vi "Email alert.vi"(6 "Email log file path":path=path "D:/3D FIB-SEM Files/Email Log", 7 "Send email":bool, 8 "Machine ID":string, 9 "Mail server":string, 10 "Alarm message":string, 11 "Recipents":string[](array[string])) -> ()   [LabVIEW 2018]
uses:
  <vilib>/Utility/SMTP/NI_SMTPEmail.lvlib
panel:
  in  "Hardware Configuration":T1={"SEM X coil"="SEM-X", "SEM Y coil"="SEM-Y", "FIB X coil"="FIB/ao0", "FIB Y coil"="FIB/ao1", "FIB Detector"="FIB/ai1", "SEM Detectors"="Detectors", "Det min (V)"=-10.0, "Det max (V)"=10.0, "Eanable COM"=TRUE, "COM port"="COM1", "FIB Beam blank"="FIB/port0/line0", "FIB Ext Scan"="FIB/port0/line1", "Det. FIB-NI auto switch"="FIB/port0/line2", "Post #1up"="Deflector/ao0", "Post #1down"="Deflector/ao1", "Post #2up"="Deflector/ao2", "Post #2down"="Deflector/ao3", "Machine Type"=0, "FIB Faraday Cup"="FIB/ai3", "Configuration file"=path "D:/Feiss.ini", "SEM Max FOV (um)"=198.5, "Machine ID"="Feiss2/Merlin-4238", "Save config file"=FALSE} {"Machine Type" items=["Feiss", "NVision"]}
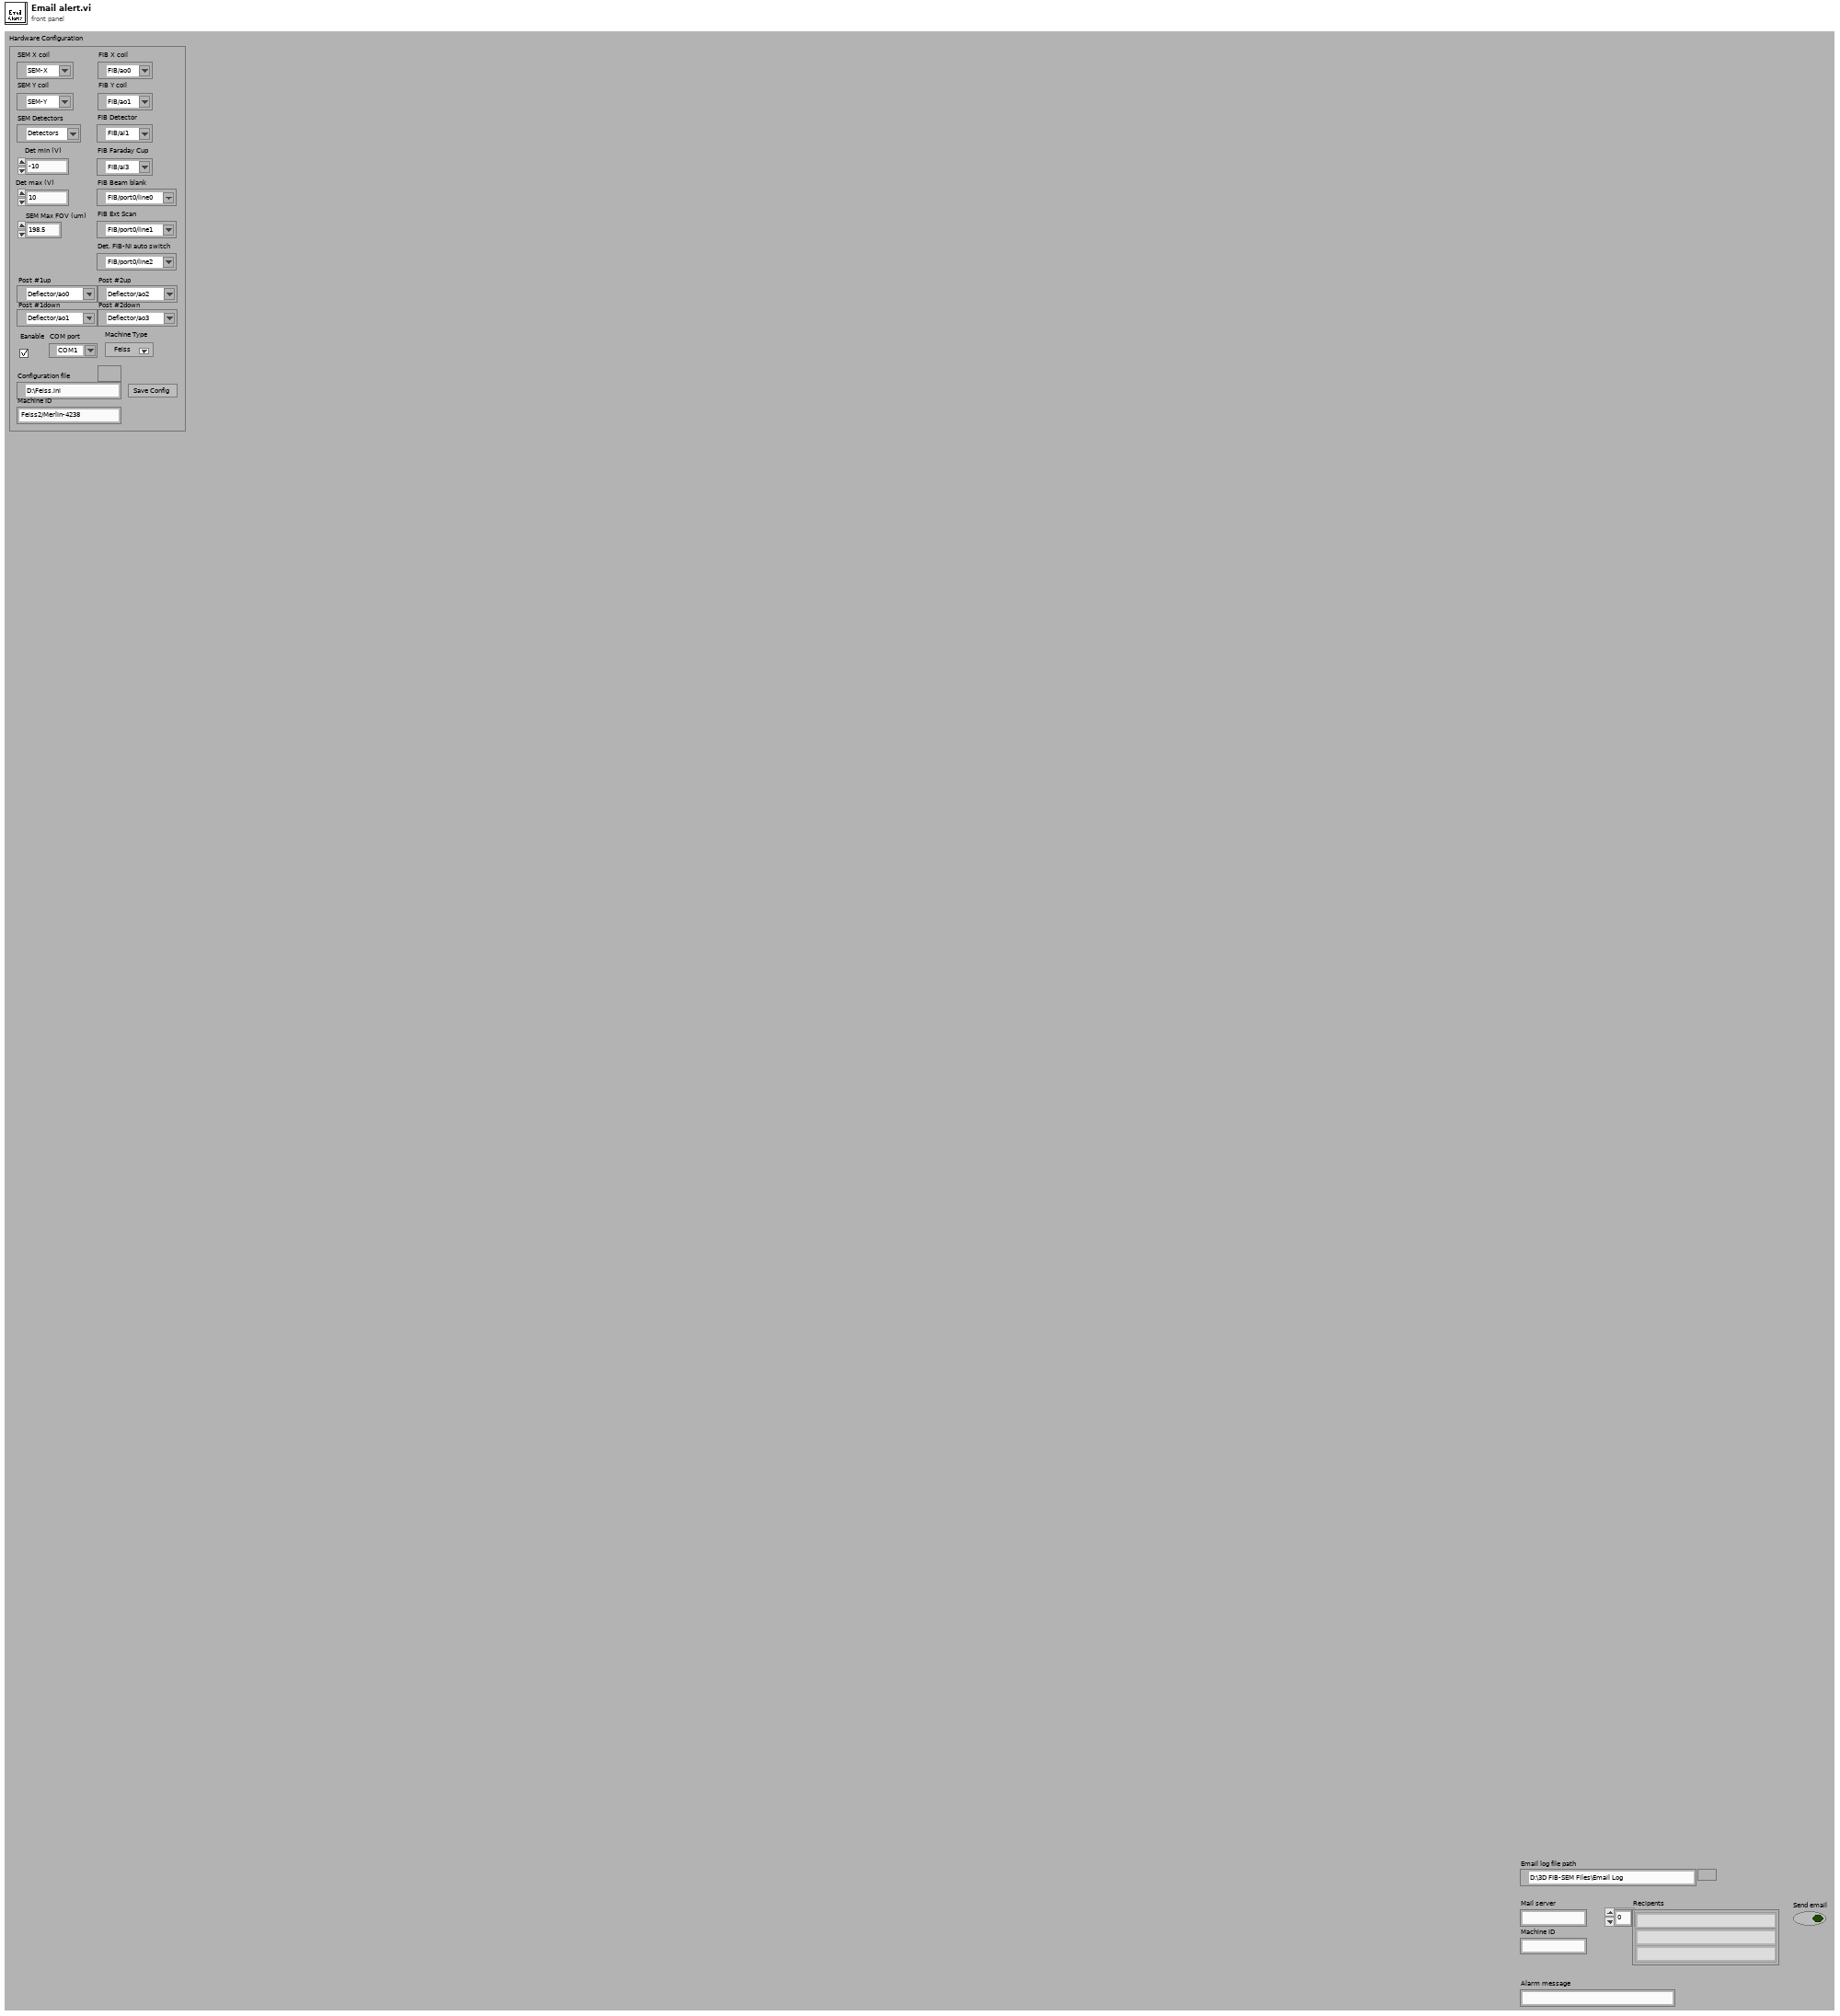
[diagram p1: front panel]
types:
  T1 = cluster{"SEM X coil":refnum<k15>, "SEM Y coil":refnum<k15>, "FIB X coil":tag, "FIB Y coil":tag, "FIB Detector":tag, "SEM Detectors":refnum<k15>, "Det min (V)":dbl, "Det max (V)":dbl, "Eanable COM":bool, "COM port":refnum<visa-resource-name>, "FIB Beam blank":tag, "FIB Ext Scan":tag, "Det. FIB-NI auto switch":tag, "Post #1up":tag, "Post #1down":tag, "Post #2up":tag, "Post #2down":tag, "Machine Type":u8, "FIB Faraday Cup":tag, "Configuration file":path, "SEM Max FOV (um)":dbl, "Machine ID":string, "Save config file":bool}
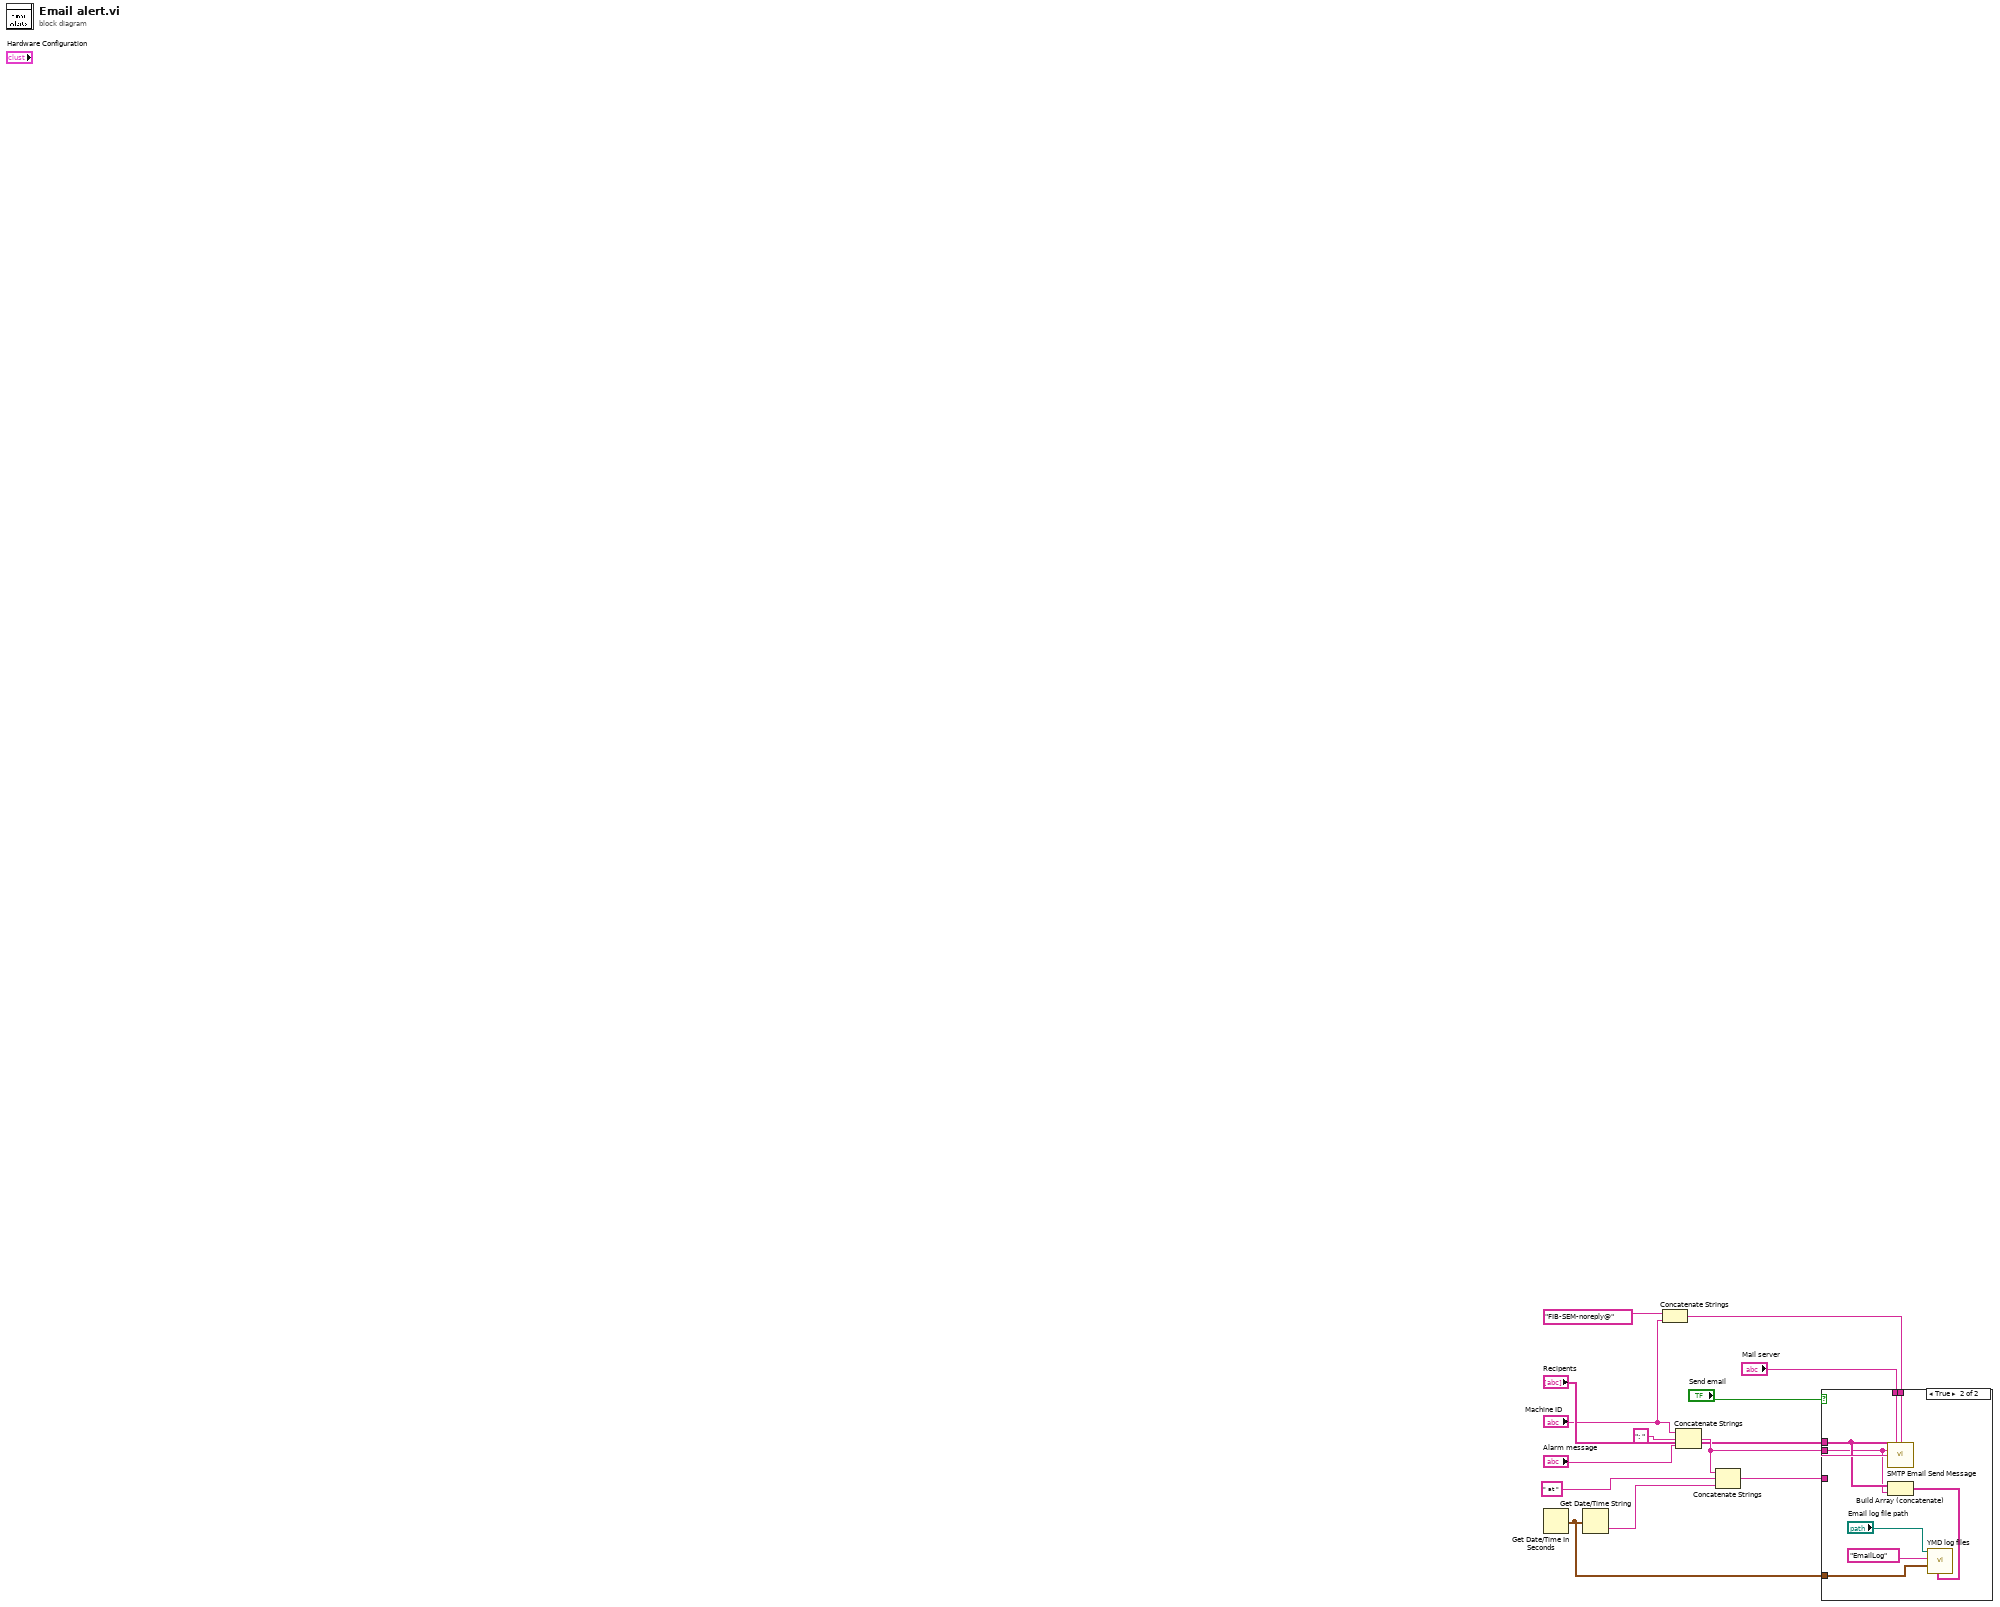
[diagram p0: block diagram]
diagram:
  n1 = Get Date/Time In Seconds() -> (seconds since 1Jan1904=w2:timestamp)
  n2 = Get Date/Time String(seconds (now)=w2) -> (time string=w1:string)  [unwired: 3 out]
  n3 = Concatenate Strings("FIB-SEM-noreply@" ("string"), "Machine ID") -> (w3:string)
  n4 = Concatenate Strings("Machine ID", ": " ("string"), "Alarm message") -> (w12:string)
  n5 = Concatenate Strings(w12, " at " ("string"), w1) -> (w13:string)
  n6 = case shown="True" "Send email" {
    tunnel: w12 -> [_ w18]
    tunnel: w13 -> [_ w22]
    tunnel: "Mail server" -> [_ w21]
    tunnel: "Recipents" -> [_ w19]
    tunnel: w3 -> [_ w20]
    tunnel: w2 -> [_ w17]
    frame False {
    }
    frame True {
      n7 = call <vilib>:"SMTP Email Send Message.vi"("recipients"=w19, "mail server"=w21, "return address"=w20, "subject ([No Subject])"=w18, "message"=w22) -> ()  [unwired: 9 in, 2 out]
      n8 = Build Array (concatenate)(w19, w18) -> (w14:string[])
      n9 = call "YMD log files.vi"("Input text array"=w14, "current time"=w17, "Log file name"="EmailLog" ("string"), "Log file path"="Email log file path") -> ()  [unwired: 8 in]
    }
  }
